vi "CRYMR_Anti_Warp_X.vi"(1 "Input":cluster{dbl, dbl}[](array[cluster]) {"?" format="%.2f"; "?" format="%.2f"}, 2 "x axis":enum32{"Linear", "Log"}(ring)) -> (0 "Output":cluster{dbl, dbl}[](array[cluster]) {"?" format="%.2f"; "?" format="%.2f"})   [LabVIEW 2013]
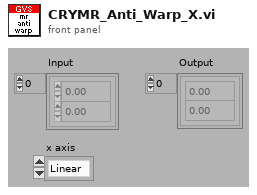
[diagram p1: front panel]
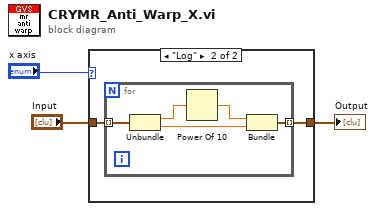
[diagram p0: block diagram]
diagram:
  n1 = case shown="\"Log\"" "x axis" {
    tunnel: "Input" -> [w4 w6]
    tunnel: [w4 w5] -> w2
    frame "Linear", Default {
    }
    frame "Log" {
      n2 = for {
        tunnel: [w11] -> w5 mode=indexing
        tunnel: w6 -> [w10] mode=indexing
        n3 = Unbundle(w10) -> (w9:dbl, w7:dbl)
        n4 = Power Of 10(x=w9) -> (10^x=w8:dbl)
        n5 = Bundle(w8, w7) -> (w11:cluster{dbl, dbl})  [unwired: 1 out]
      }
    }
  }
  "Output" <- w2
